vi "rsscope_core_global.vi"() -> ()   [LabVIEW 2014] (continued)
"Identifier"="RSSCOPE_ATTR_PMETER_MEASUREMENT_NEGATIVE_RESULT", "Descriptive Name"="Single Ended Negative Measurement Result", "Data Type"=1, "Command"="PROB{Channel}:PMET:RES:NEG?", "Access"=0, "Range Table"="", "Read Callback"="", "Write Callback"="", "Supported Models"="", "Instrument Options"="", "Flags"=0, "Help"="Returns the voltage that is measured between the negative signal socket and the ground.\n\nAvailable Repeated Capabilities:\nChannel: CH1, CH2, CH3, CH4, CHExt\r\n\nRemote-control command(s):\nPROBe<m>:PMETer:RESults:NEGative?"}, {"Level"=4, "Class Only"=FALSE, "Identifier"="RSSCOPE_ATTR_PMETER_MEASUREMENT_SINGLE_RESULT", "Descriptive Name"="Single Ended Measurement Result", "Data Type"=1, "Command"="PROB{Channel}:PMET:RES:SING?", "Access"=0, "Range Table"="", "Read Callback"="", "Write Callback"="", "Supported Models"="", "Instrument Options"="", "Flags"=0, "Help"="Returns the voltage measured between the probe tip and the ground.\n\nAvailable Repeated Capabilities:\nChannel: CH1, CH2, CH3, CH4, CHExt\r\n\nRemote-control command(s):\nPROBe<m>:PMETer:RESults:SINGle?"}, {"Level"=1, "Class Only"=TRUE, "Identifier"="", "Descriptive Name"="ZVC Probe", "Data Type"=0, "Command"="", "Access"=0, "Range Table"="", "Read Callback"="", "Write Callback"="", "Supported Models"="", "Instrument Options"="", "Flags"=0, "Help"="Contains attributes for ZVC Probe setup."}, {"Level"=2, "Class Only"=FALSE, "Identifier"="RSSCOPE_ATTR_ZVC_BANDWIDTH", "Descriptive Name"="ZVC Bandwidth", "Data Type"=1, "Command"="ZVC:BAND", "Access"=2, "Range Table"="RsScope_rngZVCBandwidth", "Read Callback"="", "Write Callback"="", "Supported Models"="", "Instrument Options"="", "Flags"=0, "Help"="Sets the bandwidth limit of the probe. The bandwidth specifies the maximum frequency at which a purely sinusoidal signal is still transferred at 89 % (0.1 dB) of its amplitude.\n\nAvailable Repeated Capabilities:\nNone\n\nRemote-control command(s):\nZVC:BANDwidth"}, {"Level"=2, "Class Only"=FALSE, "Identifier"="RSSCOPE_ATTR_ZVC_DECIMATION_MODE", "Descriptive Name"="ZVC Decimation Mode", "Data Type"=0, "Command"="ZVC:TYPE", "Access"=2, "Range Table"="RsScope_rngZVCDecimationMode", "Read Callback"="", "Write Callback"="", "Supported Models"="", "Instrument Options"="", "Flags"=0, "Help"="Sets the decimation mode for the R&S RT-ZVC probe. Decimation reduces the data stream of the ADC to a stream of waveform points with lower sample rate and a less precise time resolution.\n\nAvailable Repeated Capabilities:\nNone\n\nRemote-control command(s):\nZVC:TYPE"}, {"Level"=2, "Class Only"=FALSE, "Identifier"="RSSCOPE_ATTR_ZVC_RESOLUTION_COUPLED", "Descriptive Name"="ZVC Resolution Coupled", "Data Type"=3, "Command"="ZVC:RESC", "Access"=2, "Range Table"="", "Read Callback"="", "Write Callback"="", "Supported Models"="", "Instrument Options"="", "Flags"=0, "Help"="Sets the resolution of all R&S RT-ZVC channels. If TRUE, the resolution of the analog channels is applied to R&S RT-ZVC channels. The signal is automatically interpolated or decimated to get the analog resolution. If FALSE, the resolution of R&S RT-ZVC channels is set in a way so that the record length of the waveforms is minimum 1000 samples.\n\nAvailable Repeated Capabilities:\nNone\n\nRemote-control command(s):\nZVC:RESCoupled"}, {"Level"=2, "Class Only"=TRUE, "Identifier"="", "Descriptive Name"="ZVC Z", "Data Type"=0, "Command"="", "Access"=0, "Range Table"="", "Read Callback"="", "Write Callback"="", "Supported Models"="", "Instrument Options"="", "Flags"=0, "Help"="Contains attributes for ZVC Probe setup."}, {"Level"=3, "Class Only"=FALSE, "Identifier"="RSSCOPE_ATTR_ZVC_NAME", "Descriptive Name"="ZVC Name", "Data Type"=2, "Command"="ZVC:Z{ZVCZ}:ID:NAME?", "Access"=0, "Range Table"="", "Read Callback"="", "Write Callback"="", "Supported Models"="", "Instrument Options"="", "Flags"=0, "Help"="Queries the name of the probe.\n\nAvailable Repeated Capabilities:\nZVCZ: ZVCZ1, ZVCZ2\r\n\nRemote-control command(s):\nZVC:Z<m>:ID:NAME?"}, {"Level"=3, "Class Only"=FALSE, "Identifier"="RSSCOPE_ATTR_ZVC_PART_NUMBER", "Descriptive Name"="ZVC Part Number", "Data Type"=2, "Command"="ZVC:Z{ZVCZ}:ID:PART?", "Access"=0, "Range Table"="", "Read Callback"="", "Write Callback"="", "Supported Models"="", "Instrument Options"="", "Flags"=0, "Help"="Queries the R&S part number of the probe.\n\nAvailable Repeated Capabilities:\nZVCZ: ZVCZ1, ZVCZ2\r\n\nRemote-control command(s):\nZVC:Z<m>:ID:PARTnumber?"}, {"Level"=3, "Class Only"=FALSE, "Identifier"="RSSCOPE_ATTR_ZVC_SERIAL_NUMBER", "Descriptive Name"="ZVC Serial Number", "Data Type"=2, "Command"="ZVC:Z{ZVCZ}:ID:SRN?", "Access"=0, "Range Table"="", "Read Callback"="", "Write Callback"="", "Supported Models"="", "Instrument Options"="", "Flags"=0, "Help"="Queries the serial number of the probe.\n\nAvailable Repeated Capabilities:\nZVCZ: ZVCZ1, ZVCZ2\r\n\nRemote-control command(s):\nZVC:Z<m>:ID:SRNumber?"}, {"Level"=3, "Class Only"=FALSE, "Identifier"="RSSCOPE_ATTR_ZVC_FIRMWARE", "Descriptive Name"="ZVC Firmware", "Data Type"=2, "Command"="ZVC:Z{ZVCZ}:ID:SWV?", "Access"=0, "Range Table"="", "Read Callback"="", "Write Callback"="", "Supported Models"="", "Instrument Options"="", "Flags"=0, "Help"="Queries the version of the probe firmware.\n\nAvailable Repeated Capabilities:\nZVCZ: ZVCZ1, ZVCZ2\r\n\nRemote-control command(s):\nZVC:Z<m>:ID:SWVersion?"}, {"Level"=3, "Class Only"=TRUE, "Identifier"="", "Descriptive Name"="ZVC I", "Data Type"=0, "Command"="", "Access"=0, "Range Table"="", "Read Callback"="", "Write Callback"="", "Supported Models"="", "Instrument Options"="", "Flags"=0, "Help"="Contains attributes for ZVC Probe setup."}, {"Level"=4, "Class Only"=FALSE, "Identifier"="RSSCOPE_ATTR_ZVC_I_ENABLED", "Descriptive Name"="ZVC I Enabled", "Data Type"=3, "Command"="ZVC:Z{ZVCZ}:I{ZVCI}", "Access"=2, "Range Table"="", "Read Callback"="", "Write Callback"="", "Supported Models"="", "Instrument Options"="", "Flags"=0, "Help"="Enables the corresponding current channel of the probe.\n\nAvailable Repeated Capabilities:\nZVCZ: ZVCZ1, ZVCZ2\r\nZVCI: ZVCI1, ZVCI2, ZVCI3, ZVCI4\r\n\nRemote-control command(s):\nZVC:Z<m>:I<n>[:STATe]"}, {"Level"=4, "Class Only"=FALSE, "Identifier"="RSSCOPE_ATTR_ZVC_I_BANDWIDTH", "Descriptive Name"="ZVC I Bandwidth", "Data Type"=1, "Command"="ZVC:Z{ZVCZ}:I{ZVCI}:BAND?", "Access"=0, "Range Table"="", "Read Callback"="", "Write Callback"="", "Supported Models"="", "Instrument Options"="", "Flags"=0, "Help"="Queries the bandwidth of the current channel.\nThe bandwidth of some current channels is restricted to 300KHz due to their vertical settings.\n\nAvailable Repeated Capabilities:\nZVCZ: ZVCZ1, ZVCZ2\r\nZVCI: ZVCI1, ZVCI2, ZVCI3, ZVCI4\r\n\nRemote-control command(s):\nZVC:Z<m>:I<n>:BANDwidth?"}, {"Level"=4, "Class Only"=FALSE, "Identifier"="RSSCOPE_ATTR_ZVC_I_IMPEDANCE", "Descriptive Name"="ZVC I Impedance", "Data Type"=0, "Command"="ZVC:Z{ZVCZ}:I{ZVCI}:IMP", "Access"=2, "Range Table"="RsScope_rngZVCImpedance", "Read Callback"="", "Write Callback"="", "Supported Models"="", "Instrument Options"="", "Flags"=0, "Help"="Sets the current impedance of the probe channel for power calculations and measurements.\n\nAvailable Repeated Capabilities:\nZVCZ: ZVCZ1, ZVCZ2\r\nZVCI: ZVCI1, ZVCI2, ZVCI3, ZVCI4\r\n\nRemote-control command(s):\nZVC:Z<m>:I<n>:IMPedance"}, {"Level"=4, "Class Only"=FALSE, "Identifier"="RSSCOPE_ATTR_ZVC_I_OFFSET", "Descriptive Name"="ZVC I Offset", "Data Type"=1, "Command"="ZVC:Z{ZVCZ}:I{ZVCI}:OFFS", "Access"=2, "Range Table"="RsScope_rngZVCOffset", "Read Callback"="", "Write Callback"="", "Supported Models"="", "Instrument Options"="", "Flags"=0, "Help"="Sets the offset current for the current channel.\n\nAvailable Repeated Capabilities:\nZVCZ: ZVCZ1, ZVCZ2\r\nZVCI: ZVCI1, ZVCI2, ZVCI3, ZVCI4\r\n\nRemote-control command(s):\nZVC:Z<m>:I<n>:OFFSet"}, {"Level"=4, "Class Only"=FALSE, "Identifier"="RSSCOPE_ATTR_ZVC_I_DESKEW_OFFSET", "Descriptive Name"="ZVC I Deskew Offset", "Data Type"=1, "Command"="ZVC:Z{ZVCZ}:I{ZVCI}:SKEW", "Access"=2, "Range Table"="RsScope_rngZVCDeskewOffset", "Read Callback"="", "Write Callback"="", "Supported Models"="", "Instrument Options"="", "Flags"=0, "Help"="Sets the skew offset value for the current probe channel. This is a delay value, that is known from the circuit specifics but cannot be compensated by the instrument automatically.\n\nAvailable Repeated Capabilities:\nZVCZ: ZVCZ1, ZVCZ2\r\nZVCI: ZVCI1, ZVCI2, ZVCI3, ZVCI4\r\n\nRemote-control command(s):\nZVC:Z<m>:I<n>:SKEW"}, {"Level"=4, "Class Only"=FALSE, "Identifier"="RSSCOPE_ATTR_ZVC_I_RESET_OVERLOAD", "Descriptive Name"="ZVC I Reset Overload", "Data Type"=0, "Command"="ZVC:Z{ZVCZ}:I{ZVCI}:OVER:RSTO", "Access"=1, "Range Table"="RsScope_rngZVCResetOverload", "Read Callback"="", "Write Callback"="", "Supported Models"="", "Instrument Options"="", "Flags"=0, "Help"="Resets the overload indication at the probe.\n\nAvailable Repeated Capabilities:\nZVCZ: ZVCZ1, ZVCZ2\r\nZVCI: ZVCI1, ZVCI2, ZVCI3, ZVCI4\r\n\nRemote-control command(s):\nZVC:Z<m>:I<n>:OVERload:RSTO"}, {"Level"=4, "Class Only"=FALSE, "Identifier"="RSSCOPE_ATTR_ZVC_I_OVERLOAD_DETECTED", "Descriptive Name"="ZVC I Overload Detected", "Data Type"=3, "Command"="ZVC:Z{ZVCZ}:I{ZVCI}:OVER:VAL?", "Access"=0, "Range Table"="", "Read Callback"="", "Write Callback"="", "Supported Models"="", "Instrument Options"="", "Flags"=0, "Help"="Queries if an overload of the current channel was detected.\n\nAvailable Repeated Capabilities:\nZVCZ: ZVCZ1, ZVCZ2\r\nZVCI: ZVCI1, ZVCI2, ZVCI3, ZVCI4\r\n\nRemote-control command(s):\nZVC:Z<m>:I<n>:OVERload:VALue?"}, {"Level"=4, "Class Only"=FALSE, "Identifier"="RSSCOPE_ATTR_ZVC_I_VERTICAL_POSITION", "Descriptive Name"="ZVC I Vertical Position", "Data Type"=1, "Command"="ZVC:Z{ZVCZ}:I{ZVCI}:POS", "Access"=2, "Range Table"="RsScope_rngZVCVerticalPosition", "Read Callback"="", "Write Callback"="", "Supported Models"="", "Instrument Options"="", "Flags"=0, "Help"="Sets the vertical position of the indicated current channel as a graphical value.\n\nAvailable Repeated Capabilities:\nZVCZ: ZVCZ1, ZVCZ2\r\nZVCI: ZVCI1, ZVCI2, ZVCI3, ZVCI4\r\n\nRemote-control command(s):\nZVC:Z<m>:I<n>:POSition"}, {"Level"=4, "Class Only"=FALSE, "Identifier"="RSSCOPE_ATTR_ZVC_I_VERTICAL_SCALE", "Descriptive Name"="ZVC I Vertical Scale", "Data Type"=1, "Command"="ZVC:Z{ZVCZ}:I{ZVCI}:SCAL", "Access"=2, "Range Table"="RsScope_rngZVCVerticalScale", "Read Callback"="", "Write Callback"="", "Supported Models"="", "Instrument Options"="", "Flags"=0, "Help"="Sets the vertical scale for the current channel in Volts per division. Increasing the scale compresses the display of the signal.\n\nAvailable Repeated Capabilities:\nZVCZ: ZVCZ1, ZVCZ2\r\nZVCI: ZVCI1, ZVCI2, ZVCI3, ZVCI4\r\n\nRemote-control command(s):\nZVC:Z<m>:I<n>:SCALe"}, {"Level"=4, "Class Only"=FALSE, "Identifier"="RSSCOPE_ATTR_ZVC_I_SHUNT_MODE", "Descriptive Name"="ZVC I Shunt Mode", "Data Type"=0, "Command"="ZVC:Z{ZVCZ}:I{ZVCI}:SHUN:MODE", "Access"=2, "Range Table"="RsScope_rngZVCShuntMode", "Read Callback"="", "Write Callback"="", "Supported Models"="", "Instrument Options"="", "Flags"=0, "Help"="Sets the internal or external shunt mode.\n\nAvailable Repeated Capabilities:\nZVCZ: ZVCZ1, ZVCZ2\r\nZVCI: ZVCI1, ZVCI2, ZVCI3, ZVCI4\r\n\nRemote-control command(s):\nZVC:Z<m>:I<n>:SHUNt:MODE"}, {"Level"=4, "Class Only"=FALSE, "Identifier"="RSSCOPE_ATTR_ZVC_I_SHUNT_EXTERNAL_VALUE", "Descriptive Name"="ZVC I Shunt External Value", "Data Type"=1, "Command"="ZVC:Z{ZVCZ}:I{ZVCI}:SHUN:EVAL", "Access"=2, "Range Table"="RsScope_rngZVCShuntExternalValue", "Read Callback"="", "Write Callback"="", "Supported Models"="", "Instrument Options"="", "Flags"=0, "Help"="Defines the value of the external shunt resistor to calculate the correct current values.\n\nAvailable Repeated Capabilities:\nZVCZ: ZVCZ1, ZVCZ2\r\nZVCI: ZVCI1, ZVCI2, ZVCI3, ZVCI4\r\n\nRemote-control command(s):\nZVC:Z<m>:I<n>:SHUNt:EVALue"}, {"Level"=4, "Class Only"=FALSE, "Identifier"="RSSCOPE_ATTR_ZVC_I_SHUNT_INTERNAL_MAXIMUM", "Descriptive Name"="ZVC I Shunt Internal Maximum", "Data Type"=0, "Command"="ZVC:Z{ZVCZ}:I{ZVCI}:SHUN:MAXC", "Access"=2, "Range Table"="RsScope_rngZVCShuntIntMax", "Read Callback"="", "Write Callback"="", "Supported Models"="", "Instrument Options"="", "Flags"=0, "Help"="Sets the maximum current and the internal shunt value.\n\nAvailable Repeated Capabilities:\nZVCZ: ZVCZ1, ZVCZ2\r\nZVCI: ZVCI1, ZVCI2, ZVCI3, ZVCI4\r\n\nRemote-control command(s):\nZVC:Z<m>:I<n>:SHUNt:MAXCurrent"}, {"Level"=4, "Class Only"=FALSE, "Identifier"="RSSCOPE_ATTR_ZVC_I_SHUNT_MAXIMUM_CURRENT", "Descriptive Name"="ZVC I Shunt Maximum Current", "Data Type"=1, "Command"="ZVC:Z{ZVCZ}:I{ZVCI}:SHUN:MXCV?", "Access"=0, "Range Table"="", "Read Callback"="", "Write Callback"="", "Supported Models"="", "Instrument Options"="", "Flags"=0, "Help"="Queries the maximum current.\n\nAvailable Repeated Capabilities:\nZVCZ: ZVCZ1, ZVCZ2\r\nZVCI: ZVCI1, ZVCI2, ZVCI3, ZVCI4\r\n\nRemote-control command(s):\nZVC:Z<m>:I<n>:SHUNt:MXCValue?"}, {"Level"=4, "Class Only"=FALSE, "Identifier"="RSSCOPE_ATTR_ZVC_I_SHUNT_EXTERNAL_MAXIMUM_VOLTAGE", "Descriptive Name"="ZVC I Shunt External Maximum Voltage", "Data Type"=0, "Command"="ZVC:Z{ZVCZ}:I{ZVCI}:SHUN:MAXV", "Access"=2, "Range Table"="RsScope_rngZVCShuntExtMaxVoltage", "Read Callback"="", "Write Callback"="", "Supported Models"="", "Instrument Options"="", "Flags"=0, "Help"="Sets the maximum voltage for the external shunt.\n\nAvailable Repeated Capabilities:\nZVCZ: ZVCZ1, ZVCZ2\r\nZVCI: ZVCI1, ZVCI2, ZVCI3, ZVCI4\r\n\nRemote-control command(s):\nZVC:Z<m>:I<n>:SHUNt:MAXVoltage"}, {"Level"=4, "Class Only"=FALSE, "Identifier"="RSSCOPE_ATTR_ZVC_I_ZERO_OFFSET_DETECT", "Descriptive Name"="ZVC I Zero Offset Detect", "Data Type"=4, "Command"="ZVC:Z{ZVCZ}:I{ZVCI}:ZERC:DET", "Access"=1, "Range Table"="", "Read Callback"="", "Write Callback"="", "Supported Models"="", "Instrument Options"="", "Flags"=0, "Help"="Measures the zero offset, the mean value on a currentless DUT. If temperature changes, or if you change the shunt or other probe settings, repeat the measurement.\n\nAvailable Repeated Capabilities:\nZVCZ: ZVCZ1, ZVCZ2\r\nZVCI: ZVCI1, ZVCI2, ZVCI3, ZVCI4\r\n\nRemote-control command(s):\nZVC:Z<m>:I<n>:ZERComp:DETect"}, {"Level"=4, "Class Only"=FALSE, "Identifier"="RSSCOPE_ATTR_ZVC_I_ZERO_OFFSET_USE", "Descriptive Name"="ZVC I Zero Offset Use", "Data Type"=3, "Command"="ZVC:Z{ZVCZ}:I{ZVCI}:ZERC:USE", "Access"=2, "Range Table"="", "Read Callback"="", "Write Callback"="", "Supported Models"="", "Instrument Options"="", "Flags"=0, "Help"="Enables the automatic compensation of the measured zero offset.\n\nAvailable Repeated Capabilities:\nZVCZ: ZVCZ1, ZVCZ2\r\nZVCI: ZVCI1, ZVCI2, ZVCI3, ZVCI4\r\n\nRemote-control command(s):\nZVC:Z<m>:I<n>:ZERComp:USE"}, {"Level"=4, "Class Only"=FALSE, "Identifier"="RSSCOPE_ATTR_ZVC_I_ZERO_OFFSET_STATUS", "Descriptive Name"="ZVC I Zero Offset Status", "Data Type"=3, "Command"="ZVC:Z{ZVCZ}:I{ZVCI}:ZERC:STAT?", "Access"=0, "Range Table"="", "Read Callback"="", "Write Callback"="", "Supported Models"="", "Instrument Options"="", "Flags"=0, "Help"="Returns the status of the zero compensation of the indicated current channel.\n\nAvailable Repeated Capabilities:\nZVCZ: ZVCZ1, ZVCZ2\r\nZVCI: ZVCI1, ZVCI2, ZVCI3, ZVCI4\r\n\nRemote-control command(s):\nZVC:Z<m>:I<n>:ZERComp:STATe?"}, {"Level"=3, "Class Only"=TRUE, "Identifier"="", "Descriptive Name"="ZVC V", "Data Type"=0, "Command"="", "Access"=0, "Range Table"="", "Read Callback"="", "Write Callback"="", "Supported Models"="", "Instrument Options"="", "Flags"=0, "Help"="Contains attributes for ZVC Probe setup."}, {"Level"=4, "Class Only"=FALSE, "Identifier"="RSSCOPE_ATTR_ZVC_V_ENABLED", "Descriptive Name"="ZVC V Enabled", "Data Type"=3, "Command"="ZVC:Z{ZVCZ}:V{ZVCV}", "Access"=2, "Range Table"="", "Read Callback"="", "Write Callback"="", "Supported Models"="", "Instrument Options"="", "Flags"=0, "Help"="Enables the corresponding voltage channel of the probe.\n\nAvailable Repeated Capabilities:\nZVCZ: ZVCZ1, ZVCZ2\r\nZVCV: ZVCV1, ZVCV2, ZVCV3, ZVCV4\r\n\nRemote-control command(s):\nZVC:Z<m>:V<n>[:STATe]"}, {"Level"=4, "Class Only"=FALSE, "Identifier"="RSSCOPE_ATTR_ZVC_V_BANDWIDTH", "Descriptive Name"="ZVC V Bandwidth", "Data Type"=1, "Command"="ZVC:Z{ZVCZ}:V{ZVCV}:BAND?", "Access"=0, "Range Table"="", "Read Callback"="", "Write Callback"="", "Supported Models"="", "Instrument Options"="", "Flags"=0, "Help"="Queries the bandwidth of the voltage channel.\n\nAvailable Repeated Capabilities:\nZVCZ: ZVCZ1, ZVCZ2\r\nZVCV: ZVCV1, ZVCV2, ZVCV3, ZVCV4\r\n\nRemote-control command(s):\nZVC:Z<m>:V<n>:BANDwidth?"}, {"Level"=4, "Class Only"=FALSE, "Identifier"="RSSCOPE_ATTR_ZVC_V_IMPEDANCE", "Descriptive Name"="ZVC V Impedance", "Data Type"=0, "Command"="ZVC:Z{ZVCZ}:V{ZVCV}:IMP", "Access"=2, "Range Table"="RsScope_rngZVCImpedance", "Read Callback"="", "Write Callback"="", "Supported Models"="", "Instrument Options"="", "Flags"=0, "Help"="Sets the voltage impedance of the probe channel for power calculations and measurements.\n\nAvailable Repeated Capabilities:\nZVCZ: ZVCZ1, ZVCZ2\r\nZVCV: ZVCV1, ZVCV2, ZVCV3, ZVCV4\r\n\nRemote-control command(s):\nZVC:Z<m>:V<n>:IMPedance"}, {"Level"=4, "Class Only"=FALSE, "Identifier"="RSSCOPE_ATTR_ZVC_V_OFFSET", "Descriptive Name"="ZVC V Offset", "Data Type"=1, "Command"="ZVC:Z{ZVCZ}:V{ZVCV}:OFFS", "Access"=2, "Range Table"="RsScope_rngZVCOffset", "Read Callback"="", "Write Callback"="", "Supported Models"="", "Instrument Options"="", "Flags"=0, "Help"="Sets the vertical offset for the voltage channel.\n\nAvailable Repeated Capabilities:\nZVCZ: ZVCZ1, ZVCZ2\r\nZVCV: ZVCV1, ZVCV2, ZVCV3, ZVCV4\r\n\nRemote-control command(s):\nZVC:Z<m>:V<n>:OFFSet"}, {"Level"=4, "Class Only"=FALSE, "Identifier"="RSSCOPE_ATTR_ZVC_V_DESKEW_OFFSET", "Descriptive Name"="ZVC V Deskew Offset", "Data Type"=1, "Command"="ZVC:Z{ZVCZ}:V{ZVCV}:SKEW", "Access"=2, "Range Table"="RsScope_rngZVCDeskewOffset", "Read Callback"="", "Write Callback"="", "Supported Models"="", "Instrument Options"="", "Flags"=0, "Help"="Sets the skew offset value for the voltage probe channel. This is a delay value, that is known from the circuit specifics but cannot be compensated by the instrument automatically.\n\nAvailable Repeated Capabilities:\nZVCZ: ZVCZ1, ZVCZ2\r\nZVCV: ZVCV1, ZVCV2, ZVCV3, ZVCV4\r\n\nRemote-control command(s):\nZVC:Z<m>:V<n>:SKEW"}, {"Level"=4, "Class Only"=FALSE, "Identifier"="RSSCOPE_ATTR_ZVC_V_RESET_OVERLOAD", "Descriptive Name"="ZVC V Reset Overload", "Data Type"=4, "Command"="ZVC:Z{ZVCZ}:V{ZVCV}:OVER:RSTO", "Access"=1, "Range Table"="", "Read Callback"="", "Write Callback"="", "Supported Models"="", "Instrument Options"="", "Flags"=0, "Help"="Resets the overload indication at the probe.\n\nAvailable Repeated Capabilities:\nZVCZ: ZVCZ1, ZVCZ2\r\nZVCV: ZVCV1, ZVCV2, ZVCV3, ZVCV4\r\n\nRemote-control command(s):\nZVC:Z<m>:V<n>:OVERload:RSTO"}, {"Level"=4, "Class Only"=FALSE, "Identifier"="RSSCOPE_ATTR_ZVC_V_OVERLOAD_DETECTED", "Descriptive Name"="ZVC V Overload Detected", "Data Type"=3, "Command"="ZVC:Z{ZVCZ}:V{ZVCV}:OVER:VAL?", "Access"=0, "Range Table"="", "Read Callback"="", "Write Callback"="", "Supported Models"="", "Instrument Options"="", "Flags"=0, "Help"="Queries if an overload of the voltage channel was detected.\n\nAvailable Repeated Capabilities:\nZVCZ: ZVCZ1, ZVCZ2\r\nZVCV: ZVCV1, ZVCV2, ZVCV3, ZVCV4\r\n\nRemote-control command(s):\nZVC:Z<m>:V<n>:OVERload:VALue?"}, {"Level"=4, "Class Only"=FALSE, "Identifier"="RSSCOPE_ATTR_ZVC_V_VERTICAL_POSITION", "Descriptive Name"="ZVC V Vertical Position", "Data Type"=1, "Command"="ZVC:Z{ZVCZ}:V{ZVCV}:POS", "Access"=2, "Range Table"="RsScope_rngZVCVerticalPosition", "Read Callback"="", "Write Callback"="", "Supported Models"="", "Instrument Options"="", "Flags"=0, "Help"="Sets the vertical position of the indicated voltage channel as a graphical value.\n\nAvailable Repeated Capabilities:\nZVCZ: ZVCZ1, ZVCZ2\r\nZVCV: ZVCV1, ZVCV2, ZVCV3, ZVCV4\r\n\nRemote-control command(s):\nZVC:Z<m>:V<n>:POSition"}, {"Level"=4, "Class Only"=FALSE, "Identifier"="RSSCOPE_ATTR_ZVC_V_VERTICAL_SCALE", "Descriptive Name"="ZVC V Vertical Scale", "Data Type"=1, "Command"="ZVC:Z{ZVCZ}:V{ZVCV}:SCAL", "Access"=2, "Range Table"="RsScope_rngZVCVerticalScale", "Read Callback"="", "Write Callback"="", "Supported Models"="", "Instrument Options"="", "Flags"=0, "Help"="Sets the vertical scale for the voltage channel in Volts per division. Increasing the scale compresses the display of the signal.\n\nAvailable Repeated Capabilities:\nZVCZ: ZVCZ1, ZVCZ2\r\nZVCV: ZVCV1, ZVCV2, ZVCV3, ZVCV4\r\n\nRemote-control command(s):\nZVC:Z<m>:V<n>:SCALe"}, {"Level"=1, "Class Only"=TRUE, "Identifier"="", "Descriptive Name"="Trigger Input Probe", "Data Type"=0, "Command"="", "Access"=0, "Range Table"="", "Read Callback"="", "Write Callback"="", "Supported Models"="", "Instrument Options"="", "Flags"=0, "Help"="This class contains attributes that configure the probe on trigger input."}, {"Level"=2, "Class Only"=FALSE, "Identifier"="RSSCOPE_ATTR_TRIGGER_PROBE_STATE", "Descriptive Name"="Trigger Input Probe State", "Data Type"=0, "Command"="TRPR:SET:STAT?", "Access"=0, "Range Table"="rsscope_rngProbeState", "Read Callback"="", "Write Callback"="", "Supported Models"="", "Instrument Options"="", "Flags"=0, "Help"="Queries if the probe at the specified input channel is active (detected) or not active (not detected).\n\nAvailable Repeated Capabilities:\nNone\n\nRemote-control command(s):\nTRPRobe:SETup:STATe?"}, {"Level"=2, "Class Only"=FALSE, "Identifier"="RSSCOPE_ATTR_TRIGGER_PROBE_TYPE", "Descriptive Name"="Trigger Input Probe Type", "Data Type"=2, "Command"="TRPR:SET:TYPE?", "Access"=0, "Range Table"="", "Read Callback"="", "Write Callback"="", "Supported Models"="", "Instrument Options"="", "Flags"=0, "Help"="Queries the type of the probe.\n\nString containing one of the following values:\n None (no probe detected)\n Passive Probe\n active single-ended\n\nAvailable Repeated Capabilities:\nNone\n\nRemote-control command(s):\nTRPRobe:SETup:TYPE?"}, {"Level"=2, "Class Only"=FALSE, "Identifier"="RSSCOPE_ATTR_TRIGGER_PROBE_NAME", "Descriptive Name"="Trigger Input Probe Name", "Data Type"=2, "Command"="TRPR:SET:NAME?", "Access"=0, "Range Table"="", "Read Callback"="", "Write Callback"="", "Supported Models"="", "Instrument Options"="", "Flags"=0, "Help"="Queries the name of the probe.\n\nAvailable Repeated Capabilities:\nNone\n\nRemote-control command(s):\nTRPRobe:SETup:NAME?"}, {"Level"=2, "Class Only"=FALSE, "Identifier"="RSSCOPE_ATTR_TRIGGER_PROBE_INPUT_IMPEDANCE", "Descriptive Name"="Trigger Input Probe Input Impedance", "Data Type"=1, "Command"="TRPR:SET:IMP?", "Access"=0, "Range Table"="", "Read Callback"="", "Write Callback"="", "Supported Models"="", "Instrument Options"="", "Flags"=0, "Help"="Queries the termination of the probe.\n\nAvailable Repeated Capabilities:\nNone\n\nRemote-control command(s):\nTRPRobe:SETup:IMPedance?"}, {"Level"=2, "Class Only"=FALSE, "Identifier"="RSSCOPE_ATTR_TRIGGER_PROBE_INPUT_CAPACITANCE", "Descriptive Name"="Trigger Input Probe Input Capacitance", "Data Type"=1, "Command"="TRPR:SET:CAP?", "Access"=0, "Range Table"="", "Read Callback"="", "Write Callback"="", "Supported Models"="", "Instrument Options"="", "Flags"=0, "Help"="Queries the input capacitance of the probe.\n\nAvailable Repeated Capabilities:\nNone\n\nRemote-control command(s):\nTRPRobe:SETup:CAPacitance?"}, {"Level"=2, "Class Only"=FALSE, "Identifier"="RSSCOPE_ATTR_TRIGGER_PROBE_ATTENUATION", "Descriptive Name"="Trigger Input Probe Attenuation", "Data Type"=1, "Command"="TRPR:SET:ATT?", "Access"=0, "Range Table"="", "Read Callback"="", "Write Callback"="", "Supported Models"="", "Instrument Options"="", "Flags"=0, "Help"="Queries the attenuation of the probe.\n\nAvailable Repeated Capabilities:\nNone\n\nRemote-control command(s):\nTRPRobe:SETup:ATTenuation[:AUTO]?"}, {"Level"=2, "Class Only"=FALSE, "Identifier"="RSSCOPE_ATTR_TRIGGER_PROBE_BANDWIDTH", "Descriptive Name"="Trigger Input Probe Bandwidth", "Data Type"=1, "Command"="TRPR:SET:BAND?", "Access"=0, "Range Table"="", "Read Callback"="", "Write Callback"="", "Supported Models"="", "Instrument Options"="", "Flags"=0, "Help"="Queries the bandwidth of the probe.\n\nAvailable Repeated Capabilities:\nNone\n\nRemote-control command(s):\nTRPRobe:SETup:BANDwidth?"}, {"Level"=2, "Class Only"=FALSE, "Identifier"="RSSCOPE_ATTR_TRIGGER_PROBE_SET_OFFSET_TO_MEAN", "Descriptive Name"="Trigger Input Probe Set Offset To Mean", "Data Type"=4, "Command"="TRPR:SET:OFFS:TOM", "Access"=1, "Range Table"="", "Read Callback"="", "Write Callback"="", "Supported Models"="", "Instrument Options"="", "Flags"=1, "Help"="Sets offset to mean.\n\nAvailable Repeated Capabilities:\nNone\n\nRemote-control command(s):\nTRPRobe:SETup:OFFSet:TOMean"}, {"Level"=2, "Class Only"=FALSE, "Identifier"="RSSCOPE_ATTR_TRIGGER_PROBE_AUTO_ZERO", "Descriptive Name"="Trigger Input Probe Auto Zero", "Data Type"=4, "Command"="TRPR:SET:OFFS:AZER", "Access"=1, "Range Table"="", "Read Callback"="", "Write Callback"="", "Supported Models"="", "Instrument Options"="", "Flags"=1, "Help"="Performs an automatic correction of the zero error. If the DUT is ground-referenced, the AutoZero function can improve the measurement results.\n\nAvailable Repeated Capabilities:\nNone\n\nRemote-control command(s):\nTRPRobe:SETup:OFFSet:AZERo"}, {"Level"=2, "Class Only"=FALSE, "Identifier"="RSSCOPE_ATTR_TRIGGER_PROBE_CM_OFFSET", "Descriptive Name"="Trigger Input Probe CM Offset", "Data Type"=1, "Command"="TRPR:SET:CMOF", "Access"=2, "Range Table"="rsscope_rngProbeCMOffset", "Read Callback"="", "Write Callback"="", "Supported Models"="", "Instrument Options"="", "Flags"=0, "Help"="Sets the common-mode offset. The setting is only available for differential probes.\n\nAvailable Repeated Capabilities:\nNone\n\nRemote-control command(s):\nTRPRobe:SETup:CMOFfset"}, {"Level"=2, "Class Only"=FALSE, "Identifier"="RSSCOPE_ATTR_TRIGGER_PROBE_ATTENUATOR_ZA15", "Descriptive Name"="Trigger Input Probe Probe attenuator RT ZA15", "Data Type"=3, "Command"="TRPR:SET:ZAXV", "Access"=2, "Range Table"="", "Read Callback"="", "Write Callback"="", "Supported Models"="", "Instrument Options"="", "Flags"=0, "Help"="If you use the external attenuator R&S RT-ZA15 together with one of the differential active probes R&S RT-ZD10/20/30, enable RT-ZA15 to include the external attenuation in the measurements.\n\nAvailable Repeated Capabilities:\nNone\n\nRemote-control command(s):\nTRPRobe:SETup:ZAXV"}, {"Level"=2, "Class Only"=FALSE, "Identifier"="RSSCOPE_ATTR_TRIGGER_PROBE_MICRO_BUTTON_ACTION", "Descriptive Name"="Trigger Input Probe Micro Button Action", "Data Type"=0, "Command"="TRPR:SET:MODE", "Access"=2, "Range Table"="rsscope_rngProbeButtonAction", "Read Callback"="", "Write Callback"="", "Supported Models"="", "Instrument Options"="", "Flags"=0, "Help"="Select the action that is started with the micro button on the probe head.\n\nAvailable Repeated Capabilities:\nNone\n\nRemote-control command(s):\nTRPRobe:SETup:MODE"}, {"Level"=2, "Class Only"=FALSE, "Identifier"="RSSCOPE_ATTR_TRIGGER_PROBE_SOFTWARE_VERSION", "Descriptive Name"="Trigger Input Probe Software Version", "Data Type"=2, "Command"="TRPR:ID:SWV?", "Access"=0, "Range Table"="", "Read Callback"="", "Write Callback"="", "Supported Models"="", "Instrument Options"="", "Flags"=0, "Help"="Queries the version of the probe firmware.\n\nAvailable Repeated Capabilities:\nNone\n\nRemote-control command(s):\nTRPRobe:ID:SWVersion?"}, {"Level"=2, "Class Only"=FALSE, "Identifier"="RSSCOPE_ATTR_TRIGGER_PROBE_PRODUCTION_DATE", "Descriptive Name"="Trigger Input Probe Production Date", "Data Type"=2, "Command"="TRPR:ID:PRD?", "Access"=0, "Range Table"="", "Read Callback"="", "Write Callback"="", "Supported Models"="", "Instrument Options"="", "Flags"=0, "Help"="Queries the production date of the probe.\n\nAvailable Repeated Capabilities:\nNone\n\nRemote-control command(s):\nTRPRobe:ID:PRDate?"}, {"Level"=2, "Class Only"=FALSE, "Identifier"="RSSCOPE_ATTR_TRIGGER_PROBE_PART_NUMBER", "Descriptive Name"="Trigger Input Probe Part Number", "Data Type"=2, "Command"="TRPR:ID:PART?", "Access"=0, "Range Table"="", "Read Callback"="", "Write Callback"="", "Supported Models"="", "Instrument Options"="", "Flags"=0, "Help"="Queries the R&S part number of the probe.\n\nAvailable Repeated Capabilities:\nNone\n\nRemote-control command(s):\nTRPRobe:ID:PARTnumber?"}, {"Level"=2, "Class Only"=FALSE, "Identifier"="RSSCOPE_ATTR_TRIGGER_PROBE_SERIAL_NUMBER", "Descriptive Name"="Trigger Input Probe Serial Number", "Data Type"=2, "Command"="TRPR:ID:SRN?", "Access"=0, "Range Table"="", "Read Callback"="", "Write Callback"="", "Supported Models"="", "Instrument Options"="", "Flags"=0, "Help"="Queries the serial number of the probe.\n\nAvailable Repeated Capabilities:\nNone\n\nRemote-control command(s):\nTRPRobe:ID:SRNumber?"}, {"Level"=2, "Class Only"=FALSE, "Identifier"="RSSCOPE_ATTR_TRIGGER_PROBE_FIRMWARE_PATH", "Descriptive Name"="Trigger Input Probe Firmware Path", "Data Type"=2, "Command"="TRPR:SERV:FW:PATH", "Access"=2, "Range Table"="", "Read Callback"="", "Write Callback"="", "Supported Models"="", "Instrument Options"="", "Flags"=0, "Help"="Configures the path and file name of the update package.\n\nAvailable Repeated Capabilities:\nNone\n\nRemote-control command(s):\nTRPRobe:SERVice:FW:PATH"}, {"Level"=2, "Class Only"=FALSE, "Identifier"="RSSCOPE_ATTR_TRIGGER_PROBE_FIRMWARE_UPDATE", "Descriptive Name"="Trigger Input Probe Firmware Update", "Data Type"=4, "Command"="TRPR:SERV:FW:FLAS", "Access"=1, "Range Table"="", "Read Callback"="", "Write Callback"="", "Supported Models"="", "Instrument Options"="", "Flags"=0, "Help"="Starts the update of the probe firmware.\n\nAvailable Repeated Capabilities:\nNone\n\nRemote-control command(s):\nTRPRobe:SERVice:FW:FLASh"}, {"Level"=2, "Class Only"=FALSE, "Identifier"="RSSCOPE_ATTR_TRIGGER_PROBE_FIRMWARE_UPDATE_STATUS", "Descriptive Name"="Trigger Input Probe Firmware Update Status", "Data Type"=0, "Command"="TRPR:SERV:STAT?", "Access"=0, "Range Table"="rsscope_rngProbeFirmwareUpdateStatus", "Read Callback"="", "Write Callback"="", "Supported Models"="", "Instrument Options"="", "Flags"=0, "Help"="Queries the update status of the probe firmware.\n\nAvailable Repeated Capabilities:\nNone\n\nRemote-control command(s):\nTRPRobe:SERVice:STATe?"}, {"Level"=2, "Class Only"=FALSE, "Identifier"="RSSCOPE_ATTR_TRIGGER_PROBE_SELFTEST", "Descriptive Name"="Trigger Input Probe Selftest", "Data Type"=4, "Command"="TRPR:SERV:STES:RUN", "Access"=1, "Range Table"="", "Read Callback"="", "Write Callback"="", "Supported Models"="", "Instrument Options"="", "Flags"=0, "Help"="Starts the selftest of the probe connected to the specified channel input.\n\nAvailable Repeated Capabilities:\nNone\n\nRemote-control command(s):\nTRPRobe:SERVice:STESt:RUN"}, {"Level"=2, "Class Only"=FALSE, "Identifier"="RSSCOPE_ATTR_TRIGGER_PROBE_SELFTEST_STATUS", "Descriptive Name"="Trigger Input Probe Selftest Status", "Data Type"=0, "Command"="TRPR:SERV:STES:STAT?", "Access"=0, "Range Table"="rsscope_rngProbeSelftestStatus", "Read Callback"="", "Write Callback"="", "Supported Models"="", "Instrument Options"="", "Flags"=0, "Help"="Queries the status of a probe selftest for the specified channel input. When the selftest has finished, the status is passed or failed, otherwise it is undefined.\n\nAvailable Repeated Capabilities:\nNone\n\nRemote-control command(s):\nTRPRobe:SERVice:STESt:STATus?"}, {"Level"=2, "Class Only"=FALSE, "Identifier"="RSSCOPE_ATTR_TRIGGER_PROBE_SELFTEST_RESULT", "Descriptive Name"="Trigger Input Probe Selftest Result", "Data Type"=2, "Command"="TRPR:SERV:STES?", "Access"=0, "Range Table"="", "Read Callback"="", "Write Callback"="", "Supported Models"="", "Instrument Options"="", "Flags"=0, "Help"="Queries the status result.\n\nAvailable Repeated Capabilities:\nNone\n\nRemote-control command(s):\nTRPRobe:SERVice:STESt[:RESult]?"}, {"Level"=2, "Class Only"=FALSE, "Identifier"="RSSCOPE_ATTR_TRIGGER_PROBE_DETECTION_MODE", "Descriptive Name"="Trigger Input Probe Detection Mode", "Data Type"=0, "Command"="TRPR:SET:ATT:MODE", "Access"=2, "Range Table"="rsscope_rngAutoManual", "Read Callback"="", "Write Callback"="", "Supported Models"="", "Instrument Options"="", "Flags"=0, "Help"="Set the mode to manual if the instrument does not detect the probe.\n\nAvailable Repeated Capabilities:\nNone\n\nRemote-control command(s):\nTRPRobe:SETup:ATTenuation:MODE"}, {"Level"=2, "Class Only"=FALSE, "Identifier"="RSSCOPE_ATTR_TRIGGER_PROBE_ATTENUATION_MANUAL", "Descriptive Name"="Trigger Input Probe Attenuation Manual", "Data Type"=1, "Command"="TRPR:SET:ATT:MAN", "Access"=2, "Range Table"="rsscope_rngAttenuation", "Read Callback"="", "Write Callback"="", "Supported Models"="", "Instrument Options"="", "Flags"=0, "Help"="Sets the attenuation for the connected probe.\n\nAvailable Repeated Capabilities:\nNone\n\nRemote-control command(s):\nTRPRobe:SETup:ATTenuation:MANual"}, {"Level"=2, "Class Only"=FALSE, "Identifier"="RSSCOPE_ATTR_TRIGGER_PROBE_VERTICAL_UNIT", "Descriptive Name"="Trigger Input Probe Vertical Unit", "Data Type"=0, "Command"="TRPR:SET:ATT:UNIT", "Access"=2, "Range Table"="rsscope_rngAttUnits", "Read Callback"="", "Write Callback"="", "Supported Models"="", "Instrument Options"="", "Flags"=0, "Help"="Sets the unit for the connected probe type.\n\nAvailable Repeated Capabilities:\nNone\n\nRemote-control command(s):\nTRPRobe:SETup:ATTenuation:UNIT"}, {"Level"=2, "Class Only"=FALSE, "Identifier"="RSSCOPE_ATTR_TRIGGER_PROBE_GAIN_MANUAL", "Descriptive Name"="Trigger Input Probe Gain Manual", "Data Type"=1, "Command"="TRPR:SET:GAIN:MAN", "Access"=2, "Range Table"="rsscope_rngProbeGainManual", "Read Callback"="", "Write Callback"="", "Supported Models"="", "Instrument Options"="", "Flags"=0, "Help"="Sets the gain of a current probe.\n\nAvailable Repeated Capabilities:\nNone\n\nRemote-control command(s):\nTRPRobe:SETup:GAIN:MANual"}, {"Level"=2, "Class Only"=FALSE, "Identifier"="RSSCOPE_ATTR_TRIGGER_DETECTED_PROBE_GAIN", "Descriptive Name"="Trigger Input Detected Probe Gain", "Data Type"=1, "Command"="TRPR:SET:GAIN:AUTO?", "Access"=0, "Range Table"="", "Read Callback"="", "Write Callback"="", "Supported Models"="", "Instrument Options"="", "Flags"=0, "Help"="Returns the gain of an automatically detected current probe.\n\nAvailable Repeated Capabilities:\nNone\n\nRemote-control command(s):\nTRPRobe:SETup:GAIN:AUTO?"}, {"Level"=2, "Class Only"=FALSE, "Identifier"="RSSCOPE_ATTR_TRIGGER_PROBE_PREDEFINED_CURRENT_PROBE", "Descriptive Name"="Trigger Input Probe Predefined Current Probe", "Data Type"=0, "Command"="TRPR:SET:ATT:DEFP", "Access"=2, "Range Table"="rsscope_rngProbePredefinedCurrent", "Read Callback"="", "Write Callback"="", "Supported Models"="", "Instrument Options"="", "Flags"=0, "Help"="This attribute select the predefined current probe. Current probes are not recognized automatically but the parameters of R&S current probes (R&S RT-ZCxx) are known to the instrument.\n\nAvailable Repeated Capabilities:\nNone\n\nRemote-control command(s):\nTRPRobe:SETup:ATTenuation:DEFProbe"}, {"Level"=2, "Class Only"=FALSE, "Identifier"="RSSCOPE_ATTR_TRIGGER_INPUT_PROBE_COUPLING_AC", "Descriptive Name"="Trigger Input Probe Coupling AC", "Data Type"=3, "Command"="TRPR:SET:ACC", "Access"=2, "Range Table"="", "Read Callback"="", "Write Callback"="", "Supported Models"="", "Instrument Options"="", "Flags"=0, "Help"="Enables AC coupling in the R&S RT-ZPR20 probe, which removes DC and very low-frequency components. The R&S RT-ZPR20 probe requires 50 Ohm input termination, for which the channel AC coupling is not available. The probe setting allows AC coupling also at 50 Ohm inputs.\n\nAvailable Repeated Capabilities:\nNone\n\nRemote-control command(s):\nTRPRobe:SETup:ACCoupling"}, {"Level"=2, "Class Only"=FALSE, "Identifier"="RSSCOPE_ATTR_TRIGGER_INPUT_PROBE_RT_ZHD_OVERRANGE_BUZZER", "Descriptive Name"="Trigger Input Probe RT-ZHD Overrange Buzzer", "Data Type"=3, "Command"="TRPR:SET:ADV:AUD", "Access"=2, "Range Table"="", "Read Callback"="", "Write Callback"="", "Supported Models"="", "Instrument Options"="", "Flags"=0, "Help"="Activates the acustic overrange warning in the probe control box.\n\nAvailable Repeated Capabilities:\nNone\n\nRemote-control command(s):\nTRPRobe:SETup:ADVanced:AUDioverload"}, {"Level"=2, "Class Only"=FALSE, "Identifier"="RSSCOPE_ATTR_TRIGGER_INPUT_PROBE_RT_ZHD_BANDWIDTH_LIMIT", "Descriptive Name"="Trigger Input Probe RT-ZHD Bandwidth Limit", "Data Type"=3, "Command"="TRPR:SET:ADV:FILT", "Access"=2, "Range Table"="", "Read Callback"="", "Write Callback"="", "Supported Models"="", "Instrument Options"="", "Flags"=0, "Help"="Enables the lowpass filter in the probe control box.\n\nAvailable Repeated Capabilities:\nNone\n\nRemote-control command(s):\nTRPRobe:SETup:ADVanced:FILTer"}, {"Level"=2, "Class Only"=FALSE, "Identifier"="RSSCOPE_ATTR_TRIGGER_INPUT_PROBE_DEGAUSS", "Descriptive Name"="Trigger Input Probe Degauss", "Data Type"=4, "Command"="TRPR:SET:DEG", "Access"=1, "Range Table"="", "Read Callback"="", "Write Callback"="", "Supported Models"="", "Instrument Options"="", "Flags"=0, "Help"="Demagnetizes the core if it has been magnetized by switching the power on and off, or by an excessive input. Always carry out demagnetizing before measurement. The demagnetizing process takes about one second.\n\nAvailable Repeated Capabilities:\nNone\n\nRemote-control command(s):\nTRPRobe:SETup:DEGauss"}, {"Level"=2, "Class Only"=FALSE, "Identifier"="RSSCOPE_ATTR_TRIGGER_INPUT_PROBE_MODE", "Descriptive Name"="Trigger Input Probe Mode", "Data Type"=0, "Command"="TRPR:SET:PRM", "Access"=2, "Range Table"="RsScope_rngModularProbeMode", "Read Callback"="", "Write Callback"="", "Supported Models"="", "Instrument Options"="", "Flags"=0, "Help"="Sets the measurement mode of the modular probe.\n\nAvailable Repeated Capabilities:\nNone\n\nRemote-control command(s):\nTRPRobe:SETup:PRMode"}, {"Level"=2, "Class Only"=TRUE, "Identifier"="", "Descriptive Name"="Meter", "Data Type"=0, "Command"="", "Access"=0, "Range Table"="", "Read Callback"="", "Write Callback"="", "Supported Models"="", "Instrument Options"="", "Flags"=0, "Help"="This class contains attributes that configure the probe meter on trigger input."}, {"Level"=3, "Class Only"=FALSE, "Identifier"="RSSCOPE_ATTR_TRIGGER_PMETER_ENABLED", "Descriptive Name"="Trigger Input Probe Meter Enabled", "Data Type"=3, "Command"="TRPR:PMET:STAT", "Access"=2, "Range Table"="", "Read Callback"="", "Write Callback"="", "Supported Models"="", "Instrument Options"="", "Flags"=0, "Help"="Switches the probe meter on or off.\n\nAvailable Repeated Capabilities:\nNone\n\nRemote-control command(s):\nTRPRobe:PMETer:STATe"}, {"Level"=3, "Class Only"=FALSE, "Identifier"="RSSCOPE_ATTR_TRIGGER_PMETER_DISPLAY_DIFF", "Descriptive Name"="Trigger Display Diff", "Data Type"=0, "Command"="TRPR:SET:DISP", "Access"=2, "Range Table"="rsscope_rngProbeDisplayDiff", "Read Callback"="", "Write Callback"="", "Supported Models"="", "Instrument Options"="", "Flags"=0, "Help"="Selects the input voltages to be measured by the ProbeMeter of an R&S differential active probe.\n\nAvailable Repeated Capabilities:\nNone\n\nRemote-control command(s):\nTRPRobe:SETup:DISPlaydiff"}, {"Level"=3, "Class Only"=FALSE, "Identifier"="RSSCOPE_ATTR_TRIGGER_PMETER_VISIBILITY", "Descriptive Name"="Trigger Visibility", "Data Type"=3, "Command"="TRPR:PMET:VIS", "Access"=2, "Range Table"="", "Read Callback"="", "Write Callback"="", "Supported Models"="", "Instrument Options"="", "Flags"=0, "Help"="Activates the integrated R&S ProbeMeter of active R&S probes.\n\nAvailable Repeated Capabilities:\nNone\n\nRemote-control command(s):\nTRPRobe:PMETer:VISibility"}, {"Level"=3, "Class
